vi "Tank_Lift.vi"(11 "Drive Control":T1 {"Power (100)" min=-100 max=100}) -> ()   [LabVIEW 2012, in "Serenity_mk2.lvrbt"]
uses:
  Serenity_mk2.lvrbt
  auto_drive_TYP.ctl
  <vilib>/NXT/Hardware/Plugins/Tetrix DC Motor/TetrixDCMotorAddress.ctl
  <vilib>/NXT/NXTIO Xnodes/NXTIONodeSubVIs/TETRIX IO Move DC Motors.vi
  <vilib>/NXT/NXTIO Xnodes/NXTIONodeSubVIs/TETRIX IO Motor Status.vi
  <vilib>/NXT/NXTIO Xnodes/AddressXNode/NXTIOAddress.xnode
  <vilib>/NXT/Subs/LVHSConnector.ctl
  <vilib>/NXT/NXTIO Xnodes/NXTIOXNode/NXTIO.xnode
  <vilib>/NXT/LegoClasses/BrickReference/BrickReference.lvclass
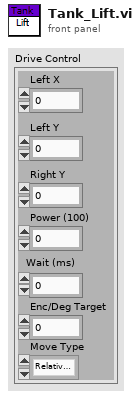
[diagram p1: front panel]
types:
  T1 = typedef "auto_drive_TYP.ctl" = cluster{"Left X":i8, "Left Y":i8, "Right Y":i8, "Power (100)":i8, "Wait (ms)":u32, "Enc/Deg Target":i32, "Move Type":enum16{"Relative Degrees", "Wait", "Encoder"}}
  T2 = typedef "TetrixDCMotorAddress.ctl" = i32
  T3 = typedef "LVHSConnector.ctl" = refnum<class "BrickReference.lvclass">
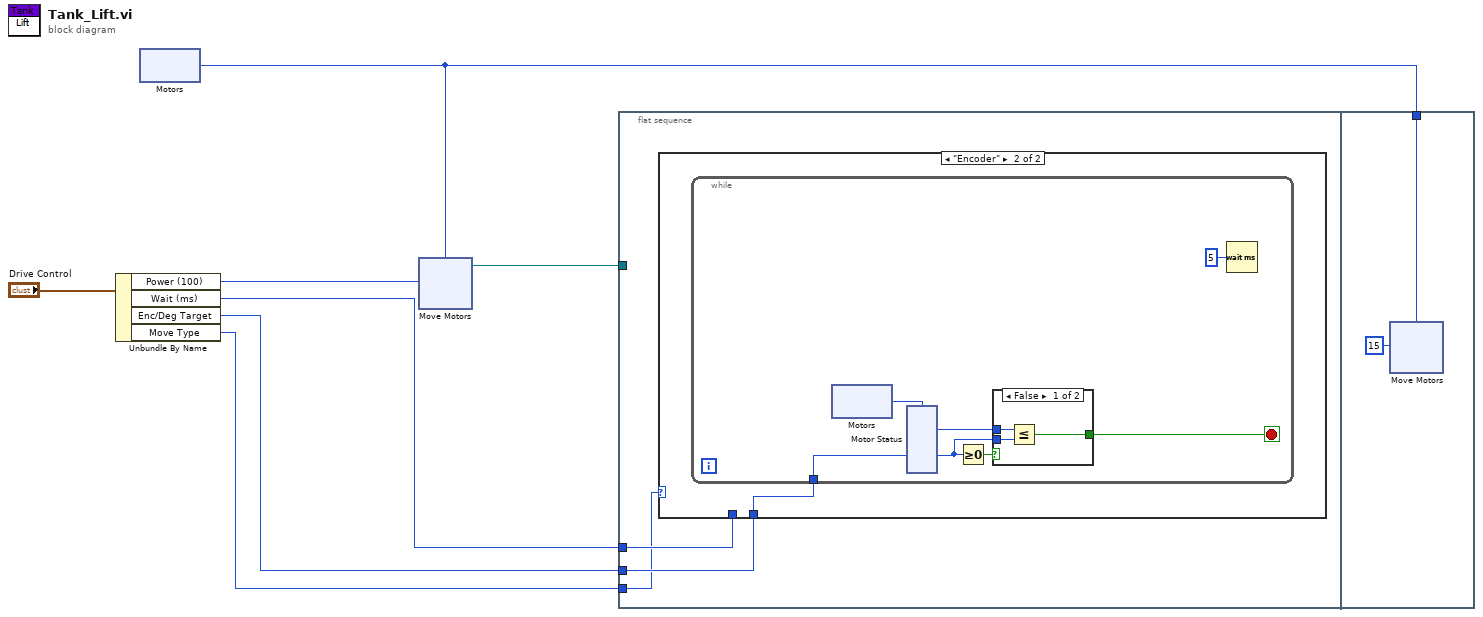
[diagram p0: block diagram]
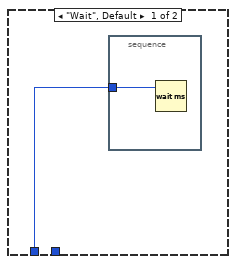
[diagram p2: hidden frame]
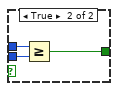
[diagram p3: hidden frame]
diagram:
  n1 = Unbundle By Name("Drive Control") -> ("Power (100)"=w3:i8, "Wait (ms)"=w5:u32, "Enc/Deg Target"=w4:i32, "Move Type"=w1:enum16{"Relative Degrees", "Wait", "Encoder"})
  n2 = xnode "Motors"() -> ("Motor"=w7:T2)
  n3 = xnode "Move Motors"("Power/Speed 1"=w3, "Motors"=w7) -> ("NXT/EV3"=w2:T3)  [unwired: 1 in]
  n4 = flat-sequence {
    tunnel: w5 -> [w10]
    tunnel: w4 -> [w9]
    tunnel: w1 -> [w8]
    tunnel: w2 -> [_]
    tunnel: w7 -> [w35]
    frame #0 {
      n5 = case shown="\"Encoder\"" w8 {
        tunnel: w10 -> [w11 _]
        tunnel: w9 -> [_ w13]
        frame "Wait", Default {
          n6 = stacked-sequence {
            tunnel: w11 -> [w12]
            frame #0 {
              n7 = Wait (ms)(milliseconds to wait=w12) -> ()  [unwired: 1 out]
            }
          }
        }
        frame "Encoder" {
          n8 = while {
            tunnel: w13 -> [w16]
            stop <- w17 stop-if-true
            n9 = xnode "Motors"() -> ("Motor"=w19:T2)
            n10 = xnode "Motor Status"("Motors"=w19) -> ("Position 1"=w15:i32)  [unwired: 1 in, 2 out]
            n11 = Greater Or Equal To 0?(x=w16) -> (x >= 0?=w18:bool)
            n12 = case shown="False" w18 {
              tunnel: w15 -> [w22 w25]
              tunnel: [w20 w24] -> w17
              tunnel: w16 -> [w21 w23]
              frame False {
                n13 = Less Or Equal?(x=w22, y=w21) -> (x <= y?=w20:bool)
              }
              frame True {
                n14 = Greater Or Equal?(x=w25, y=w23) -> (x >= y?=w24:bool)
              }
            }
            n15 = Wait (ms)(milliseconds to wait=u32 5) -> ()  [unwired: 1 out]
          }
        }
      }
    }
    frame #1 {
      n16 = xnode "Move Motors"("Power/Speed 1"=i8 15, "Motors"=w35) -> ()  [unwired: 1 in, 1 out]
    }
  }
